vi "Write SkillRef.vi"(8 "error in (no error)":errorcluster, 10 "SkillRef":refnum<class "Skill.lvclass">[](array[class]), 11 "SkillStateMachine in":refnum<class "SkillStateMachine.lvclass">) -> (0 "error out":errorcluster, 3 "SkillStateMachine out":refnum<class "SkillStateMachine.lvclass">)   [LabVIEW 2018, in "SkillStateMachine.lvclass"]
uses:
  SkillStateMachine.lvclass
  Skill_class/Skill.lvclass
  SkillStateMachine.lvclass/SkillStateMachine.ctl
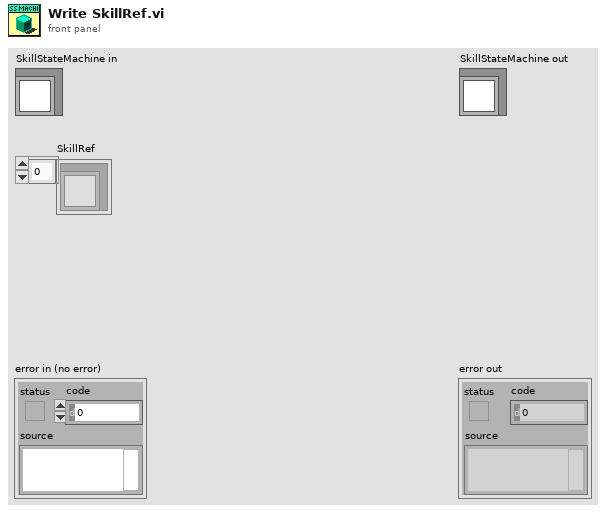
[diagram p1: front panel]
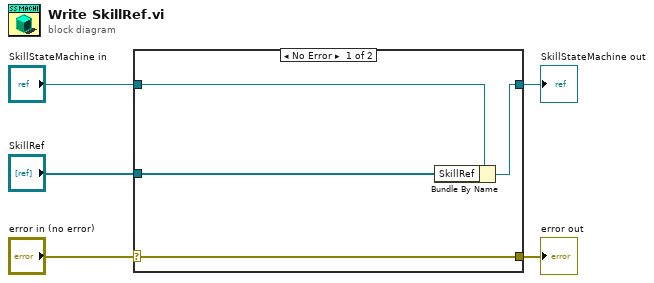
[diagram p0: block diagram]
diagram:
  n1 = case shown="No Error" "error in (no error)" {
    selector: "error in (no error)" -> [w9 w10]
    tunnel: [w9 w10] -> w4
    tunnel: [w7 w11] -> w2
    tunnel: "SkillStateMachine in" -> [w8 w11]
    tunnel: "SkillRef" -> [w6 _]
    frame No Error {
      n2 = Bundle By Name(cluster=w8, "SkillRef"=w6) -> (w7:refnum<class "SkillStateMachine.lvclass">)
    }
    frame Error {
    }
  }
  "error out" <- w4
  "SkillStateMachine out" <- w2
